vi "Test Get Failed or Not Executed Tests Filters Parameterized Skipped.vi"(11 "Result Model Result Recording Test in":refnum<class "Result Model Result Recording Test.lvclass">) -> (0 "error out":errorcluster, 3 "Result Model Result Recording Test out":refnum<class "Result Model Result Recording Test.lvclass">)   [LabVIEW 2020, in "Result Model Result Recording Test.lvclass"]
uses:
  Result Model Result Recording Test.lvclass
  C:/Program Files (x86)/National Instruments/LabVIEW 2020/vi.lib/Astemes/LUnit/Test Case.lvclass
  source/User Interface/Result Model/Tree Item Filter.ctl
  source/Core/Result/Result.ctl
  source/Core/Result/Status.ctl
  source/Core/Result/Type.ctl
  <vilib>/Astemes/LUnit/Test Case.lvclass/Test Case.ctl
  fb0f1d83-8fe4-4175-a662-44c7f83a20e6.vi
  <vilib>/Astemes/LUnit/Palette/Fail If.vi
  <vilib>/Astemes/LUnit/Core/LUnit Test Case/Private/Append Pass Result.vi
  <vilib>/Astemes/LUnit/Core/LUnit Test Case/Private/Append Fail Result.vi
  <vilib>/Astemes/LUnit/Core/LUnit Test Case/Private/Run In UI.vi
  <vilib>/Utility/error.llb/Clear Errors.vi
  source/User Interface/Result Model/Result Model.lvclass
  Result Model Result Recording Test.lvclass/Result Model Result Recording Test.ctl
  source/Core/Result/Result.lvlib
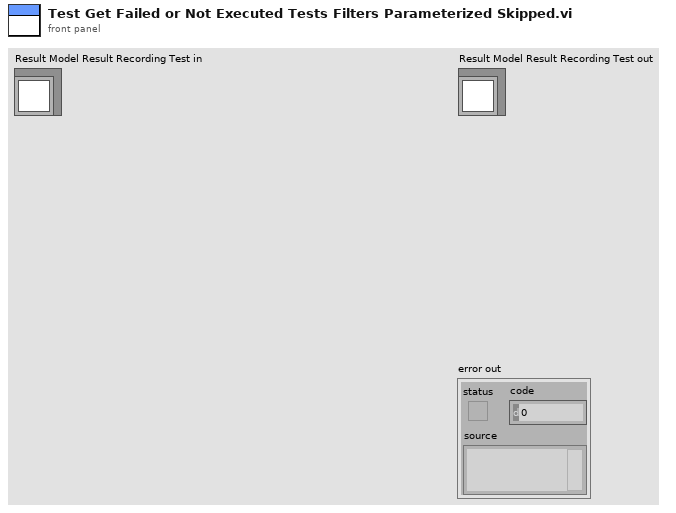
[diagram p1: front panel]
types:
  T1 = typedef "Result.lvlib/Result.ctl" = cluster{"Name":string, "Description":string, "Status":T2, "Result Type":T3, "Execution Time":dbl, "Data":cluster{"Expected":variant, "Actual":variant, "Delta":variant}}
  T2 = typedef "Result.lvlib/Status.ctl" = enum16{"", "Passed", "Failed", "Error", "Skipped", "Setup Error", "Broken", "Teardown Error"}
  T3 = typedef "Result.lvlib/Type.ctl" = enum16{"Test Case", "Test Suite", "Test Run", "Pass", "Fail", "Skip", "Pass if", "Fail if", "Pass if Error", "Fail if Error", "Pass if Equal", "Fail if Equal"}
  T4 = typedef "Result Model.lvclass/Tree Item Filter.ctl" = enum16{"All", "Only Fails", "Fails or else Not Executed"}
  T5 = cluster{"Left Cell String":string, "Child Text":string[], "Child Tag":string, "Item Indent":i32, "Child Only?":bool, "Glyph Index":i32}[]
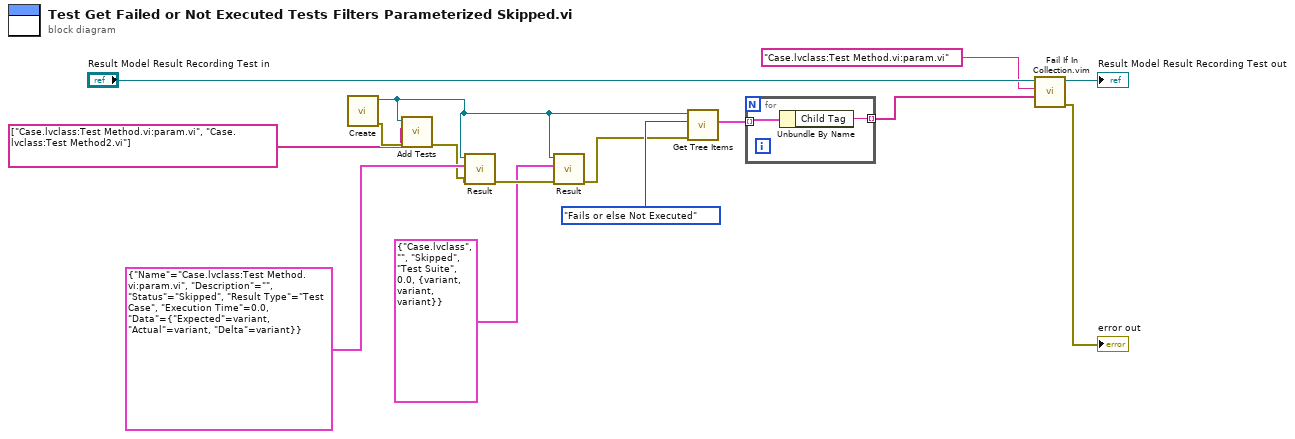
[diagram p0: block diagram]
diagram:
  n1 = call "Create.vi"() -> ("error out"=w2:errorcluster, "Result Model out"=w4:refnum<class "Result Model.lvclass">)  [unwired: 10 in]
  n2 = call "Add Tests.vi"("error in (no error)"=w2, "Tests"=string[] ["Case.lvclass:Test Method.vi:param.vi", "Case.lvclass:Test Method2.vi"], "Result Model by Reference In"=w4) -> ("error out"=w3:errorcluster)  [unwired: 8 in]
  n3 = call-dynamic "Result.vi"("error in (no error)"=w3, "Results"=T1 {"Name"="Case.lvclass:Test Method.vi:param.vi", "Description"="", "Status"=enum."Skipped", "Result Type"=enum."Test Case", "Execution Time"=0.0, "Data"={"Expected"=variant, "Actual"=variant, "Delta"=variant}}, "Result Model by Reference In"=w4) -> ("error out"=w10:errorcluster)  [unwired: 8 in]
  n4 = call-dynamic "Result.vi"("error in (no error)"=w10, "Results"=T1 {"Name"="Case.lvclass", "Description"="", "Status"=enum."Skipped", "Result Type"=enum."Test Suite", "Execution Time"=0.0, "Data"={"Expected"=variant, "Actual"=variant, "Delta"=variant}}, "Result Model by Reference In"=w4) -> ("error out"=w9:errorcluster)  [unwired: 8 in]
  n5 = call "Get Tree Items.vi"("error in (no error)"=w9, "Filter"=Tree_Item_Filter."Fails or else Not Executed", "Result Model by Reference In"=w4) -> ("Tree Items"=w6:T5)  [unwired: 7 in, 1 out]
  n6 = for {
    tunnel: w6 -> [w17] mode=indexing
    tunnel: [w16] -> w5 mode=indexing
    n7 = Unbundle By Name(w17) -> ("Child Tag"=w16:string)
  }
  n8 = call "Fail If In Collection.vim"("Collection"=w5, "Element"="Case.lvclass:Test Method.vi:param.vi" ("Name"), "LUnit Test Case In"="Result Model Result Recording Test in") -> ("error out"=→"error out":errorcluster, "LUnit Test Case Out"=→"Result Model Result Recording Test out":refnum<class "Result Model Result Recording Test.lvclass">)  [unwired: 7 in]
